vi "Destroy to Agent.vi"(8 "Error In":errorcluster, 10 "Identity":refnum<class "Agent Identity.lvclass">, 11 "Agent In":refnum<class "Agent.lvclass">) -> (0 "Error Out":errorcluster, 3 "Agent Out":refnum<class "Agent.lvclass">)   [LabVIEW 2018, in "Toolkit.lvlib" / "Agent Identity.lvclass"]
uses:
  Agent Identity.lvclass
  Agent/Agent.lvclass
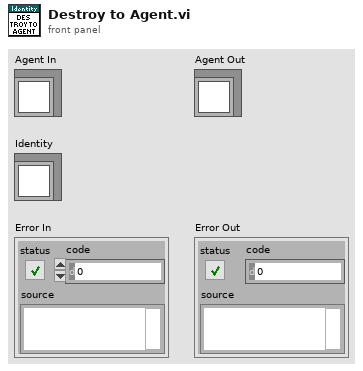
[diagram p1: front panel]
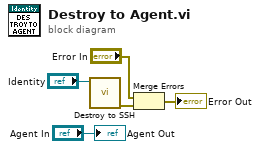
[diagram p0: block diagram]
diagram:
  n1 = call "Destroy to SSH.vi"("Identity"="Identity") -> ("Error Out"=w2:errorcluster)  [unwired: 9 in, 1 out]
  n2 = Merge Errors("Error In", w2) -> (→"Error Out":errorcluster)
  "Agent Out" <- "Agent In"
